vi "ShutDown Example.vi"() -> ()   [LabVIEW 2011, in "Messenging.lvlib"]
uses:
  Messenging.lvlib
  PP Template (Receive type)/PP Template.lvclass
  Interprocess Messenger/Send/Send.lvclass
  Interprocess Messenger/Send/Query (varients).vi
  PP Template (UserEvent).lvclass
  Parallel Process.lvclass
panel:
  out "Time":string
  in  "Event-based Active object instead of Queue-based":bool
  out "error out":errorcluster
  in  "Shutdown Method":T1(ring)
  in  "Clone if Reentrant (T)":bool=TRUE
  in  "Launch as Slave (F)":bool=TRUE
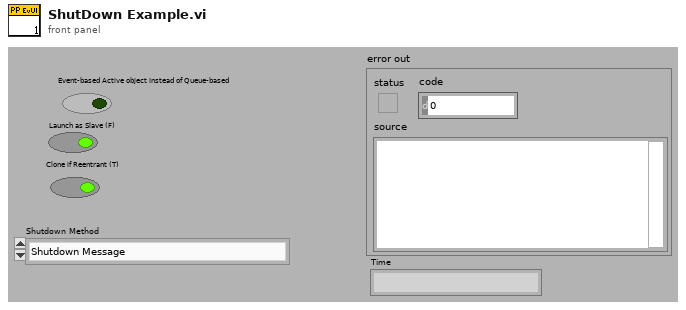
[diagram p1: front panel]
types:
  T1 = enum16{"Shutdown Message", "End Calling VI (works on Slave only)"}
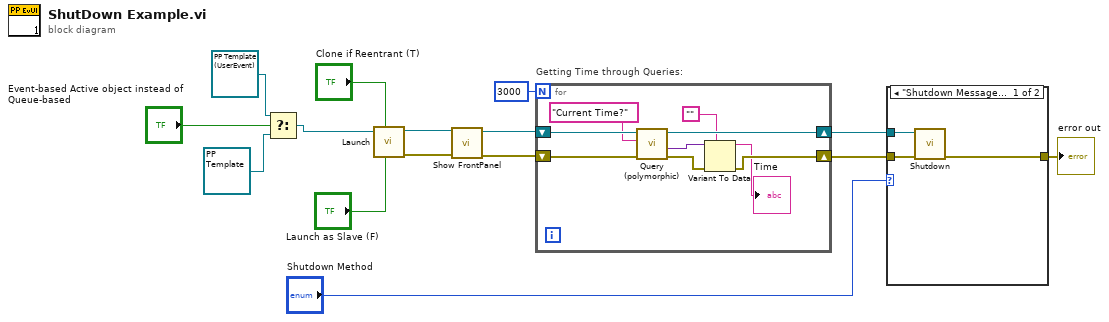
[diagram p0: block diagram]
diagram:
  n1 = Select(t=refnum<class "PP Template (UserEvent).lvclass"> refnum ("Parallel Process.lvlib:Parallel Process Template (EventUI).lvclass"), s="Event-based Active object instead of Queue-based", f=refnum<class "PP Template.lvclass"> refnum ("Messenging.lvlib:Parallel Process Template (Receive type).lvclass")) -> (s? t:f=w1:refnum<class "Parallel Process.lvclass">)
  n2 = call-dynamic "Launch.vi"("AutoShutdown Slave (F)"="Launch as Slave (F)", "Clone if Reentrant (T)"="Clone if Reentrant (T)", "Parallel Process in"=w1) -> ("error out"=w14:errorcluster, "Parallel Process out"=w15:refnum<class "Parallel Process.lvclass">)  [unwired: 1 in, 6 out]
  n3 = call-dynamic "Show FrontPanel.vi"("error in (no error)"=w14, "Parallel Process in"=w15) -> ("error out"=w10:errorcluster, "Parallel Process out"=w11:refnum<class "Parallel Process.lvclass">)  [unwired: 1 in, 7 out]
  n4 = for "Getting Time through Queries:" {
    N: 3000 -> [_]
    shift-right: [w21] -> w8
    shift-left: w11 -> [w24]
    shift-right: [w20] -> w7
    shift-left: w10 -> [w23]
    n5 = call-poly "Query (polymorphic).vi"("error in (no error)"=w23, "Label"="Current Time?", "MSR Parent"=w24) -> ("error out"=w18:errorcluster, "Replay Varient"=w19:variant, "MSR Parent"=w21:refnum<class "Parallel Process.lvclass">)  [unwired: 2 in, 4 out]
    n6 = Variant To Data(error in=w18, type="", Variant=w19) -> (data=→"Time":string, error out=w20:errorcluster)
  }
  n7 = case shown="\"Shutdown Message\"" "Shutdown Method" {
    tunnel: w8 -> [w27 _]
    tunnel: w7 -> [w26 w28]
    tunnel: [w25 w28] -> w5
    frame "Shutdown Message" {
      n8 = call-dynamic "Shutdown.vi"("error in (no error)"=w26, "Parallel Process in"=w27) -> ("error out"=w25:errorcluster)  [unwired: 2 in, 7 out]
    }
    frame "End Calling VI (works on Slave only)" {
    }
  }
  "error out" <- w5
